vi "Read Front Panel.vi"(8 "error in (no error)":errorcluster, 11 "MCListbox View in":refnum<class "MCListbox View.lvclass">) -> (0 "error out":errorcluster, 2 "Front Panel":refnum<vi>, 3 "MCListbox View out":refnum<class "MCListbox View.lvclass">)   [LabVIEW 2013, in "SET Project Editor.lvlib" / "MCListbox View.lvclass"]
uses:
  MCListbox View.lvclass
  MCListbox View.lvclass/MCListbox View.ctl
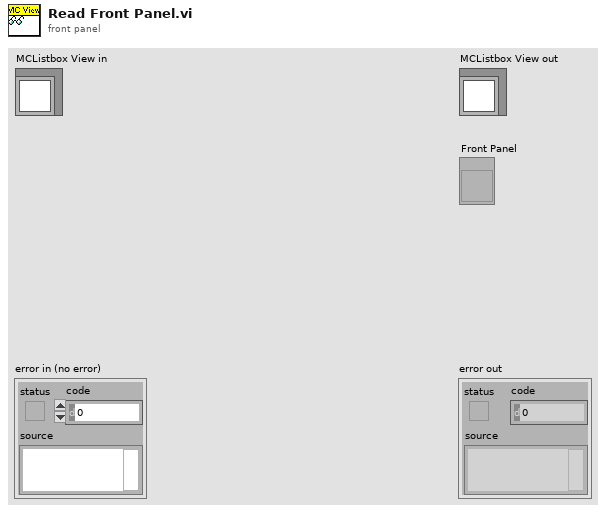
[diagram p1: front panel]
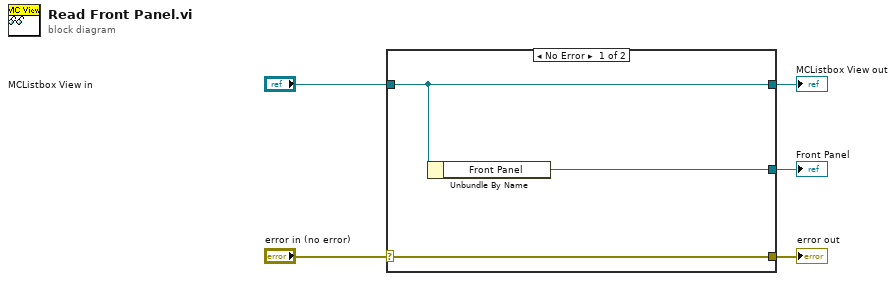
[diagram p0: block diagram]
diagram:
  n1 = case shown="No Error" "error in (no error)" {
    selector: "error in (no error)" -> [w8 w9]
    tunnel: [w8 w9] -> w4
    tunnel: [w7 w10] -> w2
    tunnel: "MCListbox View in" -> [w7 w10]
    tunnel: [w6 _] -> w1
    frame No Error {
      n2 = Unbundle By Name(w7) -> ("Front Panel"=w6:refnum<vi>)
    }
    frame Error {
    }
  }
  "error out" <- w4
  "MCListbox View out" <- w2
  "Front Panel" <- w1
